vi "Self-Test.vi"(0 "VISA resource name":refnum<visa-resource-name>, 11 "error in (no error)":errorcluster) -> (4 "VISA resource name out":refnum<visa-resource-name>, 6 "Self-Test Result Code":i32, 10 "Self-Test Result Message":string, 15 "error out":errorcluster)   [LabVIEW 2020, in "Associated Research 78XX Series.lvlib"]
doc: "Performs a self test of the instrument data memory. Returns 0 if it is successful or 1 if the test fails."
uses:
  <instrlib>/Associated Research 78XX Series/Associated Research 78XX Series.lvlib
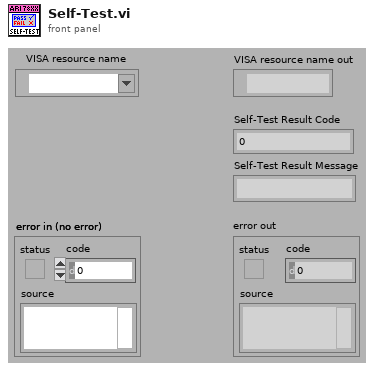
[diagram p1: front panel]
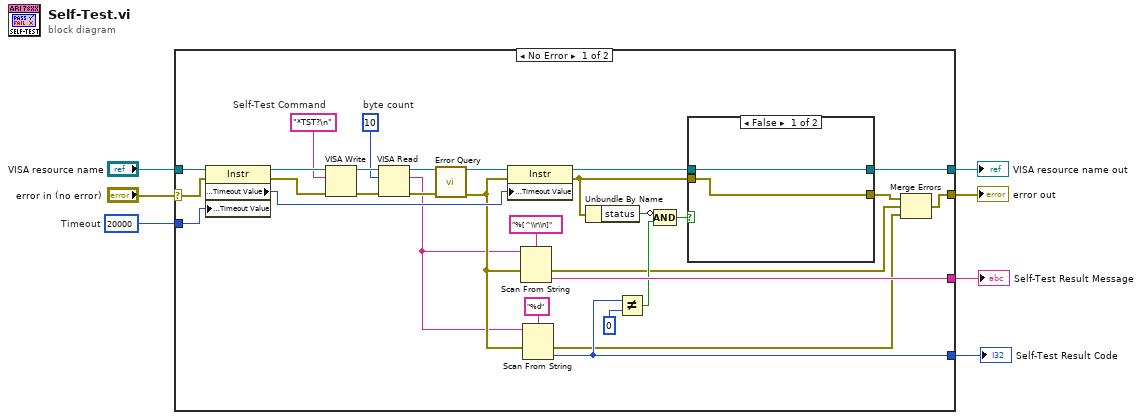
[diagram p0: block diagram]
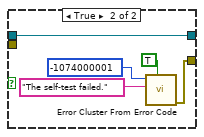
[diagram p2: hidden frame]
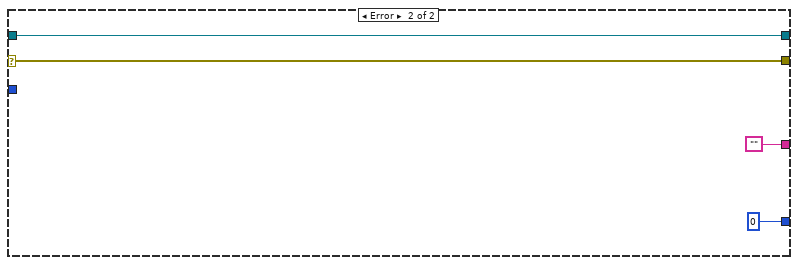
[diagram p3: hidden frame]
diagram:
  w3 = u32 20000  # Timeout
  n1 = case shown="No Error" "error in (no error)" {
    selector: "error in (no error)" -> [w18 w47]
    tunnel: "VISA resource name" -> [w33 w48]
    tunnel: [w13 w48] -> w6
    tunnel: [w14 w47] -> w5
    tunnel: [w31 "" ("Empty String Constant")] -> w4
    tunnel: w3 -> [w30 _]
    tunnel: [w20 0] -> w2
    frame No Error {
      w32 = u32 10  # byte count
      w26 = "*TST?\n"  # Self-Test Command
      n2 = property on="Property Node" class="Instr"(reference=w33, error in=w18, "General Settings:Timeout Value"=w30) -> (reference out=w28:refnum<visa-resource-name>, error out=w29:errorcluster, "General Settings:Timeout Value"=w27:u32)
      n3 = VISA Write(VISA resource name=w28, write buffer=w26, error in (no error)=w29) -> (VISA resource name out=w35:refnum<visa-resource-name>, error out=w34:errorcluster)  [unwired: 1 out]
      n4 = VISA Read(VISA resource name=w35, byte count=w32, error in (no error)=w34) -> (VISA resource name out=w12:refnum<visa-resource-name>, read buffer=w8:string, error out=w11:errorcluster)  [unwired: 1 out]
      n5 = call <instrlib>:"Error Query.vi"("VISA resource name"=w12, "error in (no error)"=w11) -> ("VISA resource name out"=w10:refnum<visa-resource-name>, "error out"=w9:errorcluster)  [unwired: 10 in, 2 out]
      n6 = property on="Property Node" class="Instr"(reference=w10, error in=w9, "General Settings:Timeout Value"=w27) -> (reference out=w25:refnum<visa-resource-name>, error out=w24:errorcluster)
      n7 = Scan From String(format string="%[^\\r\\n]" ("Format String"), input string=w8, error in=w9) -> (error out=w15:errorcluster, output 1=w31:string)  [unwired: 2 in, 2 out]
      n8 = Scan From String(format string="%d", input string=w8, error in=w9) -> (error out=w16:errorcluster, output 1=w20:i32)  [unwired: 2 in, 2 out]
      n9 = Unbundle By Name(w24) -> ("status"=w22:bool)
      n10 = Not Equal?(x=w20, y=0) -> (x != y?=w23:bool)
      n11 = Compound Arithmetic op=AND(invert w22, w23) -> (w21:bool)
      n12 = case shown="False" w21 {
        tunnel: w25 -> [w39 w44]
        tunnel: w24 -> [w38 _]
        tunnel: [w38 w40] -> w17
        tunnel: [w39 w44] -> w13
        frame False {
        }
        frame True {
          n13 = call <vilib>:"Error Cluster From Error Code.vi"("show call chain? (False)"=TRUE, "error message (\"\")"="The self-test failed." ("Source (VI Name)"), "error code (0)"=-1074000001 ("Code")) -> ("error out"=w40:errorcluster)  [unwired: 6 in]
        }
      }
      n14 = Merge Errors(w17, w15, w16) -> (w14:errorcluster)
    }
    frame Error {
    }
  }
  "Self-Test Result Message" <- w4
  "Self-Test Result Code" <- w2
  "VISA resource name out" <- w6
  "error out" <- w5
